vi "Ex3Task3end.vi"() -> ()   [LabVIEW 2014, in "Ex3Task2.lvrbt"]
uses:
  Ex3Task2.lvrbt
panel:
  out "Moving Average":dbl
  out "Random Number":dbl
  in  "stop":bool
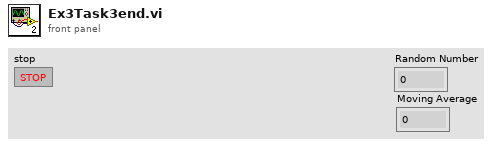
[diagram p1: front panel]
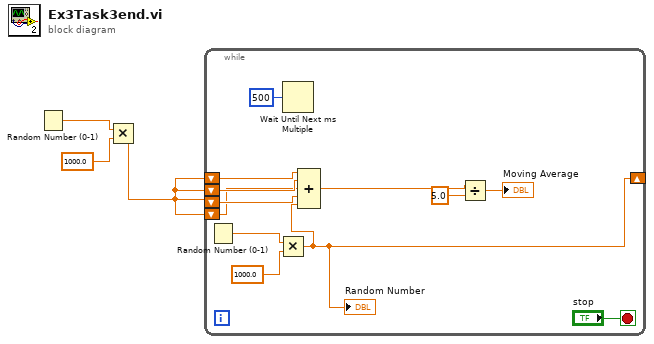
[diagram p0: block diagram]
diagram:
  n1 = Random Number (0-1)() -> (number: 0 to 1=w3:dbl)
  n2 = Multiply(x=w3, y=1000.0) -> (x*y=w1:dbl)
  n3 = while {
    shift-right: [w4] -> _
    shift-left: w1 -> [w12]
    shift-left: w1 -> [w11]
    shift-left: w1 -> [w10]
    shift-left: w1 -> [w5]
    stop <- "stop" stop-if-true
    n4 = Random Number (0-1)() -> (number: 0 to 1=w15:dbl)
    n5 = Multiply(x=w15, y=1000.0) -> (x*y=w4:dbl)
    "Random Number" <- w4
    n6 = Wait Until Next ms Multiple(millisecond multiple=u32 500) -> ()  [unwired: 1 out]
    n7 = Compound Arithmetic op=ADD(w12, w11, w5, w10, w4) -> (w8:dbl)
    n8 = Divide(x=w8, y=5.0) -> (x/y=→"Moving Average":dbl)
  }
